vi "Set Type Descriptor.vi"(8 "error in (no error)":errorcluster, 10 "Type Descriptor":T1={"Name"="", "Direction"=enum."Sink", "Value Type"=enum."Bool", "Default"=variant, "Terminal Mode"=enum."Recommended", "Min"=variant, "Max"=variant, "Step"=variant, "Options"=[], "Terminal Type"=enum."Unwired", "Type Mode"=enum."Output", "Value Mode"=enum."Basic"}, 11 "Type Descriptor in":refnum<class "Type Descriptor.lvclass">) -> (0 "error out":errorcluster, 3 "Type Descriptor out":refnum<class "Type Descriptor.lvclass">)   [LabVIEW 2020, in "Parallel Block.lvlib" / "Type Descriptor.lvclass"]
uses:
  Type Descriptor.lvclass
  Type Descriptor.ctl
  Direction.ctl
  Value Type.ctl
  Terminal Mode.ctl
  Terminal Type.ctl
  Type Descriptor.lvclass/Type Descriptor.ctl
  Parallel Block.lvlib
  Type Mode.ctl
  Value Mode.ctl
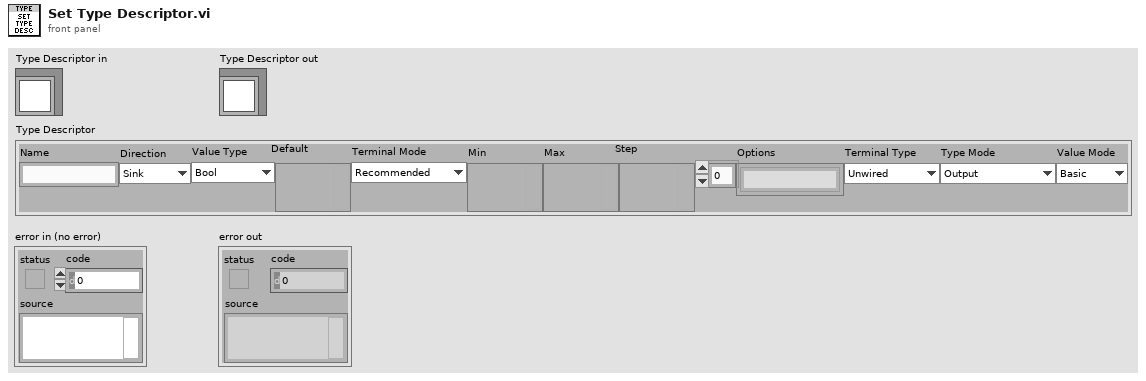
[diagram p1: front panel]
types:
  T1 = typedef "Parallel Block.lvlib/Type Descriptor.ctl" = cluster{"Name":string, "Direction":T2, "Value Type":T3, "Default":variant, "Terminal Mode":T4, "Min":variant, "Max":variant, "Step":variant, "Options":string[], "Terminal Type":T5, "Type Mode":T6, "Value Mode":T7}
  T2 = typedef "Parallel Block.lvlib/Direction.ctl" = enum16{"Sink", "Source"}
  T3 = typedef "Parallel Block.lvlib/Value Type.ctl" = enum16{"Unknown", "Bool", "U8", "U16", "U32", "U64", "I8", "I16", "I32", "I64", "SGL", "DBL", "CSG", "CDB", "CDBWfm", "String", "DBLWfm"}
  T4 = typedef "Parallel Block.lvlib/Terminal Mode.ctl" = enum16{"Recommended", "Required", "None"}
  T5 = typedef "Parallel Block.lvlib/Terminal Type.ctl" = enum16{"Unwired", "BadType", "Connection", "Value", "Control Ref", "BadRefType"}
  T6 = typedef "Parallel Block.lvlib/Type Mode.ctl" = enum16{"Output", "Adaptive (Lossy)", "Strict (Lossy)", "Lossless"}
  T7 = typedef "Parallel Block.lvlib/Value Mode.ctl" = enum16{"Basic", "Range", "Select"}
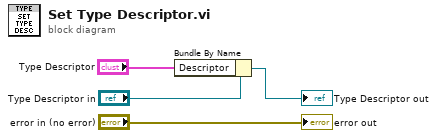
[diagram p0: block diagram]
diagram:
  n1 = Bundle By Name(cluster="Type Descriptor in", "Descriptor"="Type Descriptor") -> (→"Type Descriptor out":refnum<class "Type Descriptor.lvclass">)
  "error out" <- "error in (no error)"
